vi "ArmGoToPosition.vi"(0 "RobotConfig":T6={"Motors"={"DriveLeftPrimary"={"CAN Address"=1, "Invert"=FALSE, "InvertSensor"=FALSE, "Unit Conversion Factor"=0.0, "Brake Mode"=enum."Override to Brake", "Reverse Limt Switch Mode"=enum."Normally Closed", "Forward Limt Swith Mode"=enum."Normally Closed"}, "DriveLeftSecondary1"={"CAN Address"=2, "Invert"=FALSE, "InvertSensor"=FALSE, "Unit Conversion Factor"=0.0, "Brake Mode"=enum."Override to Brake", "Reverse Limt Switch Mode"=enum."Normally Closed", "Forward Limt Swith Mode"=enum."Normally Closed"}, "DriveRightPrimary"={"CAN Address"=3, "Invert"=FALSE, "InvertSensor"=FALSE, "Unit Conversion Factor"=0.0, "Brake Mode"=enum."Override to Brake", "Reverse Limt Switch Mode"=enum."Normally Closed", "Forward Limt Swith Mode"=enum."Normally Closed"}, "DriveRightSecondary1"={"CAN Address"=4, "Invert"=FALSE, "InvertSensor"=FALSE, "Unit Conversion Factor"=0.0, "Brake Mode"=enum."Override to Brake", "Reverse Limt Switch Mode"=enum."Normally Closed", "Forward Limt Swith Mode"=enum."Normally Closed"}, "RightIntake"={"CAN Address"=8, "Invert"=FALSE, "InvertSensor"=FALSE, "Unit Conversion Factor"=0.0, "Brake Mode"=enum."Override to Brake", "Reverse Limt Switch Mode"=enum."Normally Closed", "Forward Limt Swith Mode"=enum."Normally Closed"}, "LeftIntake"={"CAN Address"=7, "Invert"=FALSE, "InvertSensor"=FALSE, "Unit Conversion Factor"=0.0, "Brake Mode"=enum."Override to Brake", "Reverse Limt Switch Mode"=enum."Normally Closed", "Forward Limt Swith Mode"=enum."Normally Closed"}, "ArmPivot"={"CAN Address"=5, "Invert"=FALSE, "InvertSensor"=FALSE, "Unit Conversion Factor"=0.0, "Brake Mode"=enum."Override to Brake", "Reverse Limt Switch Mode"=enum."Normally Closed", "Forward Limt Swith Mode"=enum."Normally Closed"}, "ArmExtend"={"CAN Address"=6, "Invert"=FALSE, "InvertSensor"=FALSE, "Unit Conversion Factor"=0.0, "Brake Mode"=enum."Override to Brake", "Reverse Limt Switch Mode"=enum."Normally Closed", "Forward Limt Swith Mode"=enum."Normally Closed"}, "ArmPivot2"={"CAN Address"=9, "Invert"=FALSE, "InvertSensor"=FALSE, "Unit Conversion Factor"=0.0, "Brake Mode"=enum."Override to Brake", "Reverse Limt Switch Mode"=enum."Normally Closed", "Forward Limt Swith Mode"=enum."Normally Closed"}, "Climber"={"CAN Address"=10, "Invert"=FALSE, "InvertSensor"=FALSE, "Unit Conversion Factor"=0.0, "Brake Mode"=enum."Override to Brake", "Reverse Limt Switch Mode"=enum."Disabled", "Forward Limt Swith Mode"=enum."Disabled"}}, "Sensors"={"IMU"={"Yaw Axis"=enum."Z", "SPI Bus"=enum."SPI MXP", "AHRS Algorithm"=enum."Complementary", "Calibration Time (s)"=3.0, "Calibrate On Open"=TRUE}, "LimitSwitch1"={"DIOChannel"=enum."DIO 0", "Active Low"=FALSE}, "LimitSwitch2"={"DIOChannel"=enum."DIO 1", "Active Low"=FALSE}, "BeamBreak"={"DIOChannel"=enum."DIO 2", "Active Low"=FALSE}, "JeVois"={"Baud Rate"=9600, "Parity"=0, "Data Bits"=8, "Stop Bits"=10, "Termination Char (0xA = '\\n' = LF)"=10, "Enable Termination Char? (T)"=TRUE, "Flow Control"=0, "Timeout Value (ms)"=5000, "Serial Port"=enum."Onboard RS-232"}}, "PID"={"ArmExtend"={"P"=0.0, "I"=0.0, "D"=0.0, "F"=0.0, "IZone"=0.0}, "ArmRotate"={"P"=0.0, "I"=0.0, "D"=0.0, "F"=0.0, "IZone"=0.0}, "Drive"={"P"=0.0, "I"=0.0, "D"=0.0, "F"=0.0, "IZone"=0.0}, "DriveGyro Kp ((in/sec)/deg)"=0.0}, "Solenoids"={"ArmClaw"={"Forward Channel"=enum."Solenoid 0", "Invert"=FALSE, "Reverse Channel"=enum."Solenoid 0"}, "IntakeExtend"={"Forward Channel"=enum."Solenoid 1", "Invert"=FALSE, "Reverse Channel"=enum."Solenoid 0"}, "IntakeOpen"={"Forward Channel"=enum."Solenoid 2", "Invert"=FALSE, "Reverse Channel"=enum."Solenoid 0"}, " Shifter"={"Forward Channel"=enum."Solenoid 3", "Invert"=FALSE, "Reverse Channel"=enum."Solenoid 0"}}, "RobotDimensions "={"Length"=0.0, "Height"=0.0, "HeightOfBumpers"=0.0, "DistanceFromFrameEdgeToPyramid "=0.0, "HeightOfFrameToIntake"=0.0, "EdgeOfFrameToOrigin"=0.0}, "ArmHomePosition"={"Angle (rad)"=0.0, "Radius (in)"=0.0}} {"Sensors"."JeVois"."Flow Control" items=["None", "XON/XOFF", "RTS/CTS", "XON/XOFF & RTS/CTS", "DTR/DSR", "XON/XOFF & DTR/DSR"]; "Sensors"."JeVois"."Termination Char (0xA = '\\n' = LF)" format="%.0x"; "Sensors"."JeVois"."Stop Bits" items=["1.0"=10, "1.5"=15, "2.0"=20]; "Sensors"."JeVois"."Parity" items=["None", "Odd", "Even", "Mark", "Space"]}, 1 "ArmPlanRequest":T1, 2 "Arm min Extension (in)":dbl, 3 "Arm max Extension (in)":dbl, 4 "Arm positions":T28, 5 "Avoidance Polygon":T26, 6 "Arm extend motor":T21={"DeviceStatus"={"status"=FALSE, "code"=0, "source"=""}, "Type"=enum."PWM", "PWM"={"PWM Channel"=enum."Invalid", "DeadBand"={"Name"="", "maxPositivePwm"=0, "minPositivePwm"=0, "centerPwm"=0, "maxNegativePwm"=0, "minNegativePwm"=0, "angularRange"=0}}, "CAN"={"Device Number"=0, "SetOutput VI Ref"=variant(enum8{"Percent VBus", "Current", "Speed", "Position", "Voltage"} enum."Percent VBus"), "GetOutput VI Ref"=variant(refnum<k1> refnum), "Enable VI Ref"=variant(dbl 12.0), "Disable VI Ref"=variant(enum8{"Percent VBus", "Speed", "Position", "Slave", "Unchanged / Invalid", "Voltage Compensation", "Current", "Motion Profile"} enum."Percent VBus"), "Data"=variant}, "Invert"=FALSE, "DIO PWM"={"PWM \"Enable\" Channel"=enum."Invalid", "DIOChannel"=enum."Invalid", "PWM Rate"=0.0}}, 7 "MotionProfileGeneratorParameters":T25={"Trajectory Point Interval (ms)"=10, "Maximum Travel Speed (units/s)"=0.0, "Velocity Ramp Time (ms)"=0.0, "Acceleration Ramp Time (ms)"=1.0} {"Acceleration Ramp Time (ms)" min=1.0; "Velocity Ramp Time (ms)" min=1.0; "Maximum Travel Speed (units/s)" min=0.0; "Trajectory Point Interval (ms)" items=["TrajectoryDuration_0ms"=0, "TrajectoryDuration_5ms"=5, "TrajectoryDuration_10ms"=10, "TrajectoryDuration_20ms"=20, "TrajectoryDuration_30ms"=30, "TrajectoryDuration_40ms"=40, "TrajectoryDuration_50ms"=50, "TrajectoryDuration_100ms"=100]}, 8 "Arm rotate motor":T21={"DeviceStatus"={"status"=FALSE, "code"=0, "source"=""}, "Type"=enum."PWM", "PWM"={"PWM Channel"=enum."Invalid", "DeadBand"={"Name"="", "maxPositivePwm"=0, "minPositivePwm"=0, "centerPwm"=0, "maxNegativePwm"=0, "minNegativePwm"=0, "angularRange"=0}}, "CAN"={"Device Number"=0, "SetOutput VI Ref"=variant(enum8{"Percent VBus", "Current", "Speed", "Position", "Voltage"} enum."Percent VBus"), "GetOutput VI Ref"=variant(refnum<k1> refnum), "Enable VI Ref"=variant(dbl 12.0), "Disable VI Ref"=variant(enum8{"Percent VBus", "Speed", "Position", "Slave", "Unchanged / Invalid", "Voltage Compensation", "Current", "Motion Profile"} enum."Percent VBus"), "Data"=variant}, "Invert"=FALSE, "DIO PWM"={"PWM \"Enable\" Channel"=enum."Invalid", "DIOChannel"=enum."Invalid", "PWM Rate"=0.0}}) -> (14 "ArmPlanResponse":T3 {"ExtendTrajectory"."Time (ms)" items=["TrajectoryDuration_0ms"=0, "TrajectoryDuration_5ms"=5, "TrajectoryDuration_10ms"=10, "TrajectoryDuration_20ms"=20, "TrajectoryDuration_30ms"=30, "TrajectoryDuration_40ms"=40, "TrajectoryDuration_50ms"=50, "TrajectoryDuration_100ms"=100]; "RotateTrajectory"."Time (ms)" items=["TrajectoryDuration_0ms"=0, "TrajectoryDuration_5ms"=5, "TrajectoryDuration_10ms"=10, "TrajectoryDuration_20ms"=20, "TrajectoryDuration_30ms"=30, "TrajectoryDuration_40ms"=40, "TrajectoryDuration_50ms"=50, "TrajectoryDuration_100ms"=100]})   [LabVIEW 2017]
uses:
  TypeDefs/ArmPositions.ctl
  General/PathPlanning/TypeDefs/Point2D.ctl
  General/PathPlanning/TypeDefs/Polygon2D.ctl
  General/MotionProfiling/TypeDefs/MotionProfileGeneratorParams.ctl
  <vilib>/Rock Robotics/WPI/ThirdParty/Phoenix-LabVIEW/Motor Controller/Controls/CTRE_Phoenix_MotorControl_TrajectoryPointTimeDur.ctl
  <vilib>/Rock Robotics/WPI/MotorControl/WPI_MotorControlDeviceRef.ctl
  <vilib>/Rock Robotics/WPI/MotorControl/WPI_MotorControlType.ctl
  <vilib>/Rock Robotics/SystemInterfaces/DIO/FPGA_DIOPWMChannel.ctl
  <vilib>/Rock Robotics/WPI/PWM/WPI_PWMDeadband.ctl
  <vilib>/Rock Robotics/SystemInterfaces/DIO/FPGA_DIOChannel.ctl
  TypeDefs/ConfigComponents/Config_Robot.ctl
  TypeDefs/ConfigComponents/Config_Motor.ctl
  <vilib>/Rock Robotics/WPI/ThirdParty/Phoenix-LabVIEW/Motor Controller/Controls/CTRE_Phoenix_MotorControl_NeutralMode.ctl
  <vilib>/Rock Robotics/WPI/ThirdParty/Phoenix-LabVIEW/Motor Controller/Controls/CTRE_Phoenix_MotorControl_LimitSwitchNormal.ctl
  TypeDefs/ConfigComponents/Config_IMU.ctl
  <vilib>/Rock Robotics/SystemInterfaces/spilib/spi_bus.ctl
  TypeDefs/ConfigComponents/Config_DigitalIO.ctl
  TypeDefs/ConfigComponents/Config_SerialPort.ctl
  <vilib>/Rock Robotics/WPI/SerialPort/WPI_SerialPort.ctl
  TypeDefs/ConfigComponents/Config_PIDParams.ctl
  TypeDefs/ConfigComponents/Config_DoubleSolenoid.ctl
  <vilib>/Rock Robotics/WPI/Solenoid/WPI_SolenoidChannel.ctl
  TypeDefs/ConfigComponents/Config_Dimensions.ctl
  TypeDefs/ConfigComponents/Config_ArmHome.ctl
  TypeDefs/ArmPlanResponse.ctl
  General/MotionProfiling/TypeDefs/TrajectoryPoint.ctl
  TypeDefs/ArmPlanRequest.ctl
  TypeDefs/ArmTargetPosition.ctl
  <vilib>/Rock Robotics/WPI/ThirdParty/Phoenix-LabVIEW/Motor Controller/Get/CTRE_Phoenix_MotorController_GetSelectedSensorData.vi
  Global_Var-RefNum/LEDData.vi
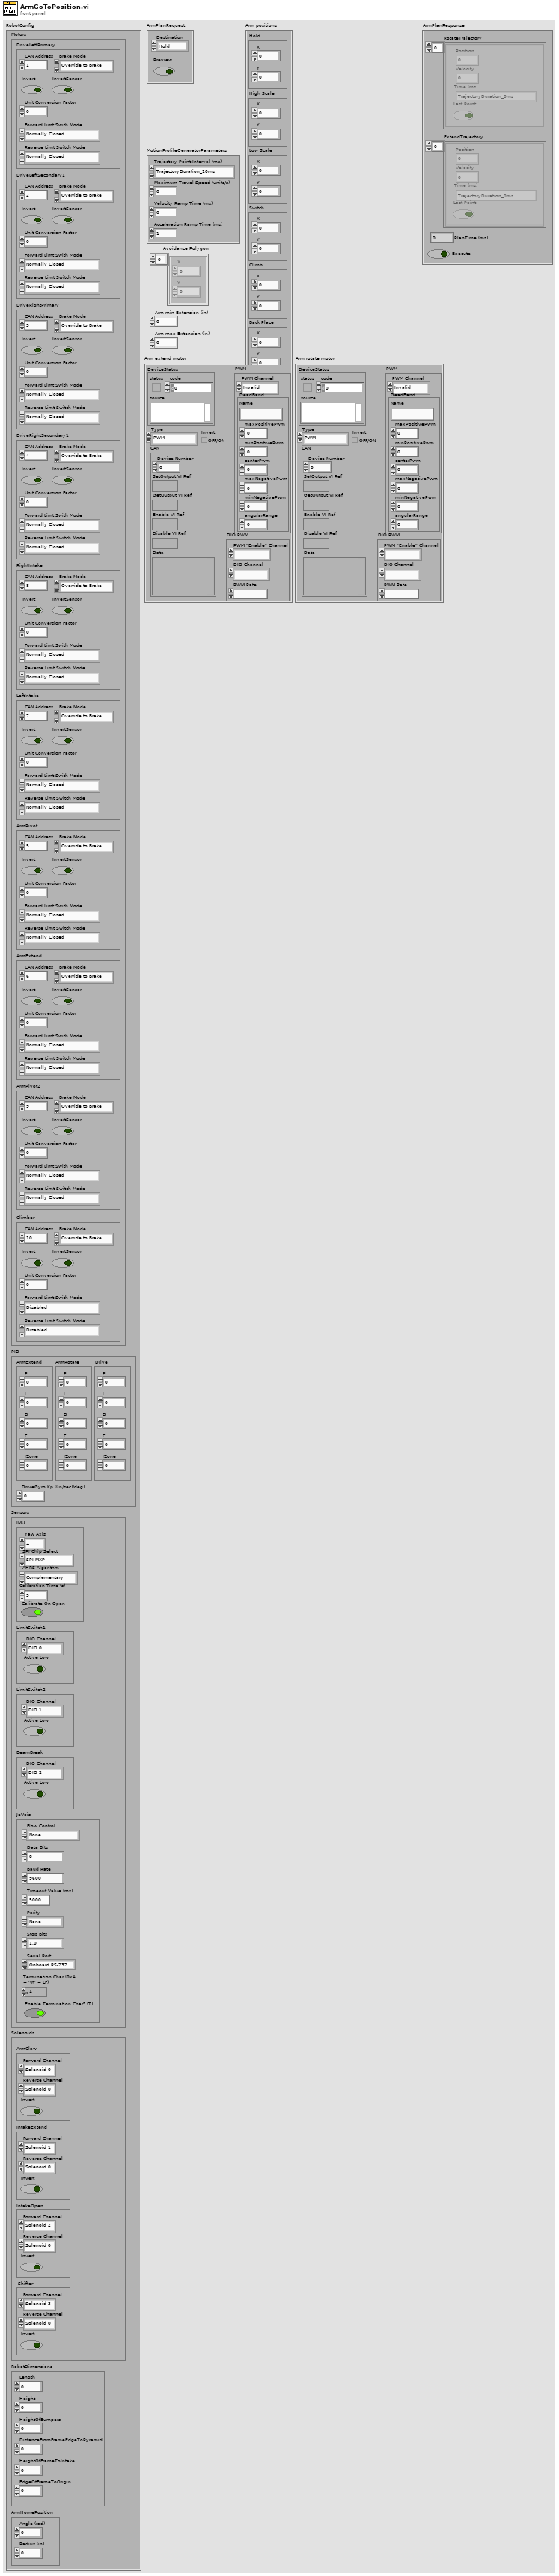
[diagram p1: front panel]
types:
  T1 = typedef "ArmPlanRequest.ctl" = cluster{"Destination":T2, "Preview":bool}
  T2 = typedef "ArmTargetPosition.ctl" = enum16{"Hold", "Switch", "Scale Low", "Scale High", "Climb", "Back Place"}
  T3 = typedef "ArmPlanResponse.ctl" = cluster{"RotateTrajectory":T4[], "ExtendTrajectory":T4[], "PlanTime (ms)":u32, "Execute":bool}
  T4 = typedef "TrajectoryPoint.ctl" = cluster{"Position ":dbl, "Velocity ":dbl, "Time (ms)":T5, "Last Point":bool}
  T5 = typedef "CTRE_Phoenix_MotorControl_TrajectoryPointTimeDur.ctl" = i32
  T6 = typedef "Config_Robot.ctl" = cluster{"Motors":cluster{"DriveLeftPrimary":T7, "DriveLeftSecondary1":T7, "DriveRightPrimary":T7, "DriveRightSecondary1":T7, "RightIntake":T7, "LeftIntake":T7, "ArmPivot":T7, "ArmExtend":T7, "ArmPivot2":T7, "Climber":T7}, "Sensors":cluster{"IMU":T10, "LimitSwitch1":T12, "LimitSwitch2":T12, "BeamBreak":T12, "JeVois":T14}, "PID":cluster{"ArmExtend":T16, "ArmRotate":T16, "Drive":T16, "DriveGyro Kp ((in/sec)/deg)":dbl}, "Solenoids":cluster{"ArmClaw":T17, "IntakeExtend":T17, "IntakeOpen":T17, " Shifter":T17}, "RobotDimensions ":T19, "ArmHomePosition":T20}
  T7 = typedef "Config_Motor.ctl" = cluster{"CAN Address":u8, "Invert":bool, "InvertSensor":bool, "Unit Conversion Factor":dbl, "Brake Mode":T8, "Reverse Limt Switch Mode":T9, "Forward Limt Swith Mode":T9}
  T8 = typedef "CTRE_Phoenix_MotorControl_NeutralMode.ctl" = enum8{"EEPROMSetting", "Override to Coast", "Override to Brake"}
  T9 = typedef "CTRE_Phoenix_MotorControl_LimitSwitchNormal.ctl" = enum16{"Normally Open", "Normally Closed", "Disabled"}
  T10 = typedef "Config_IMU.ctl" = cluster{"Yaw Axis":enum16{"X", "Y", "Z"}, "SPI Bus":T11, "AHRS Algorithm":enum16{"Complementary", "Madgwick"}, "Calibration Time (s)":dbl, "Calibrate On Open":bool}
  T11 = typedef "spi_bus.ctl" = enum16{"SPI On-Board, CS0", "SPI On-Board, CS1", "SPI On-Board, CS2", "SPI On-Board, CS3", "SPI MXP", "Invalid"}
  T12 = typedef "Config_DigitalIO.ctl" = cluster{"DIOChannel":T13, "Active Low":bool}
  T13 = typedef "FPGA_DIOChannel.ctl" = enum8{"DIO 0", "DIO 1", "DIO 2", "DIO 3", "DIO 4", "DIO 5", "DIO 6", "DIO 7", "DIO 8", "DIO 9", "DIO MXP 0", "DIO MXP 1", "DIO MXP 2", "DIO MXP 3", "DIO MXP 4", "DIO MXP 5", "DIO MXP 6", "DIO MXP 7", "DIO MXP 8", "DIO MXP 9", "DIO MXP 10", "DIO MXP 11", "DIO MXP 12", "DIO MXP 13", "DIO MXP 14", "DIO MXP 15", "SPI Port CS1", "SPI Port CS2", "SPI Port CS3", "SPI Port MISO", "SPI Port MOSI", "Invalid"}
  T14 = typedef "Config_SerialPort.ctl" = cluster{"Baud Rate":u32, "Parity":u16, "Data Bits":u16, "Stop Bits":u16, "Termination Char (0xA = '\\n' = LF)":u8, "Enable Termination Char? (T)":bool, "Flow Control":u16, "Timeout Value (ms)":u32, "Serial Port":T15}
  T15 = typedef "WPI_SerialPort.ctl" = enum16{"Onboard RS-232", "MXP TTL", "USB 1", "USB 2"}
  T16 = typedef "Config_PIDParams.ctl" = cluster{"P":dbl, "I":dbl, "D":dbl, "F":dbl, "IZone":dbl}
  T17 = typedef "Config_DoubleSolenoid.ctl" = cluster{"Forward Channel":T18, "Invert":bool, "Reverse Channel":T18}
  T18 = typedef "WPI_SolenoidChannel.ctl" = enum8{"Solenoid 0", "Solenoid 1", "Solenoid 2", "Solenoid 3", "Solenoid 4", "Solenoid 5", "Solenoid 6", "Solenoid 7", "Invalid"}
  T19 = typedef "Config_Dimensions.ctl" = cluster{"Length":dbl, "Height":dbl, "HeightOfBumpers":dbl, "DistanceFromFrameEdgeToPyramid ":dbl, "HeightOfFrameToIntake":dbl, "EdgeOfFrameToOrigin":dbl}
  T20 = typedef "Config_ArmHome.ctl" = cluster{"Angle (rad)":dbl, "Radius (in)":dbl}
  T21 = typedef "WPI_MotorControlDeviceRef.ctl" = cluster{"DeviceStatus":errorcluster, "Type":T22, "PWM":cluster{"PWM Channel":T23, "DeadBand":T24}, "CAN":cluster{"Device Number":u8, "SetOutput VI Ref":variant, "GetOutput VI Ref":variant, "Enable VI Ref":variant, "Disable VI Ref":variant, "Data":variant}, "Invert":bool, "DIO PWM":cluster{"PWM \"Enable\" Channel":T23, "DIOChannel":T13, "PWM Rate":dbl}}
  T22 = typedef "WPI_MotorControlType.ctl" = enum16{"PWM", "CAN", "DIO PWM"}
  T23 = typedef "FPGA_DIOPWMChannel.ctl" = enum8{"PWM 0", "PWM 1", "PWM 2", "PWM 3", "PWM 4", "PWM 5", "PWM 6", "PWM 7", "PWM 8", "PWM 9", "PWM MXP 0", "PWM MXP 1", "PWM MXP 2", "PWM MXP 3", "PWM MXP 4", "PWM MXP 5", "PWM MXP 6", "PWM MXP 7", "PWM MXP 8", "PWM MXP 9", "Invalid"}
  T24 = typedef "WPI_PWMDeadband.ctl" = cluster{"Name":string, "maxPositivePwm":i32, "minPositivePwm":i32, "centerPwm":i32, "maxNegativePwm":i32, "minNegativePwm":i32, "angularRange":u16}
  T25 = typedef "MotionProfileGeneratorParams.ctl" = cluster{"Trajectory Point Interval (ms)":T5, "Maximum Travel Speed (units/s)":dbl, "Velocity Ramp Time (ms)":dbl, "Acceleration Ramp Time (ms)":dbl}
  T26 = typedef "Polygon2D.ctl" = T27[]
  T27 = typedef "Point2D.ctl" = cluster{"X":dbl, "Y":dbl}
  T28 = typedef "ArmPositions.ctl" = cluster{"Hold":T27, "High Scale":T27, "Low Scale":T27, "Switch":T27, "Climb":T27, "Back Place":T27}
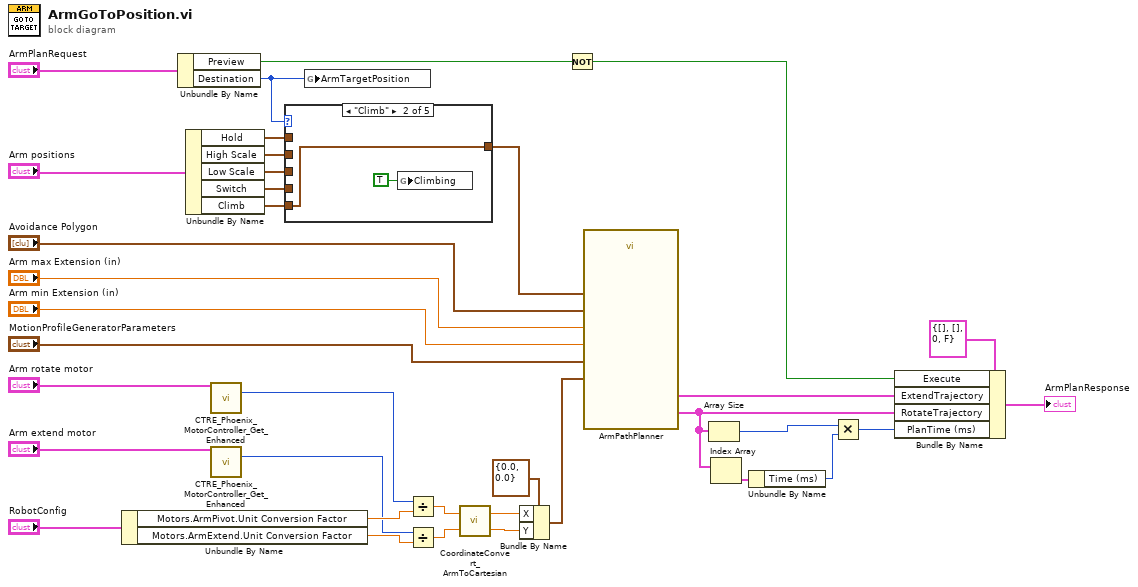
[diagram p0: block diagram]
diagram:
  n1 = Unbundle By Name("RobotConfig") -> ("Motors.ArmPivot.Unit Conversion Factor"=w29:dbl, "Motors.ArmExtend.Unit Conversion Factor"=w27:dbl)
  n2 = Unbundle By Name("ArmPlanRequest") -> ("Preview"=w10:bool, "Destination"=w1:T2)
  n3 = Unbundle By Name("Arm positions") -> ("Hold"=w4:T27, "High Scale"=w5:T27, "Low Scale"=w6:T27, "Switch"=w7:T27, "Climb"=w9:T27)
  n4 = call-poly <vilib>:"CTRE_Phoenix_MotorController_Get_Enhanced.vi"("PhoenixMotorControlDevRef"="Arm rotate motor") -> ("Position (Raw Sensor Units)"=w28:i32)  [unwired: 11 in, 3 out]
  n5 = call-poly <vilib>:"CTRE_Phoenix_MotorController_Get_Enhanced.vi"("PhoenixMotorControlDevRef"="Arm extend motor") -> ("Position (Raw Sensor Units)"=w26:i32)  [unwired: 11 in, 3 out]
  n6 = case shown="\"Climb\"" w1 {
    tunnel: w9 -> [_ w39 _ _ _]
    tunnel: [w37 w39 w40 w41 w42] -> w8
    tunnel: w7 -> [_ _ w40 _ _]
    tunnel: w6 -> [_ _ _ w41 _]
    tunnel: w5 -> [_ _ _ _ w42]
    tunnel: w4 -> [w37 _ _ _ _]
    frame "Hold", Default {
    }
    frame "Climb" {
      n7 = global write "LEDData.vi" "Climbing"(TRUE ("Climbing")) -> ()
    }
    frame "Switch" {
    }
    frame "Scale Low" {
    }
    frame "Scale High" {
    }
  }
  n8 = global write "LEDData.vi" "ArmTargetPosition"(w1) -> ()
  n9 = Divide(x=w28, y=w29) -> (x/y=w25:dbl)
  n10 = Divide(x=w26, y=w27) -> (x/y=w24:dbl)
  n11 = call "CoordinateConvert_ArmToCartesian.vi"("Radius (in)"=w24, "Angle (rad)"=w25) -> ("Y (in)"=w21:dbl, "X (in)"=w22:dbl)
  n12 = Bundle By Name(cluster=T27 {"X"=0.0, "Y"=0.0} ("2DPoint"), "X"=w22, "Y"=w21) -> (w20:T27)
  n13 = Not(x=w10) -> (.not. x?=w2:bool)
  n14 = call "ArmPathPlanner.vi"("StartPoint"=w20, "EndPoint"=w8, "MinArmLength"="Arm min Extension (in)", "MaxArmLength"="Arm max Extension (in)", "AvoidancePolygon"="Avoidance Polygon", "MotionProfileGeneratorParameters"="MotionProfileGeneratorParameters") -> ("RotatePath"=w16:T4[], "ExtendPath"=w17:T4[])  [unwired: 10 in, 2 out]
  n15 = Array Size(array=w16) -> (size(s)=w14:i32)
  n16 = Index Array(array=w16) -> (element=w15:T4)  [unwired: 1 in]
  n17 = Unbundle By Name(w15) -> ("Time (ms)"=w13:T5)
  n18 = Multiply(x=w14, y=w13) -> (x*y=w12:T5)
  n19 = Bundle By Name(cluster=T3 {"RotateTrajectory"=[], "ExtendTrajectory"=[], "PlanTime (ms)"=0, "Execute"=FALSE} ("ArmPlanResponse"), "Execute"=w2, "ExtendTrajectory"=w17, "RotateTrajectory"=w16, "PlanTime (ms)"=w12) -> (→"ArmPlanResponse":T3)
